vi "Set Options.vi"(8 "error in (no error)":errorcluster, 10 "UI Options":T1, 11 "FormulaG API in":refnum<class "FormulaG API.lvclass">) -> (0 "error out":errorcluster, 3 "FormulaG API out":refnum<class "FormulaG API.lvclass">)   [LabVIEW 2020, in "FormulaG.lvlib" / "FormulaG API.lvclass"]
uses:
  FormulaG API.lvclass
  FormulaG-Common/UI Options.ctl
  Command.ctl
  FormulaG API.lvclass/FormulaG API.ctl
  <vilib>/IlluminatedG/IG GodotServer/GodotLV/GodotServer/GodotServer.lvclass
  FormulaG-Common/FormulaG-Common.lvlib
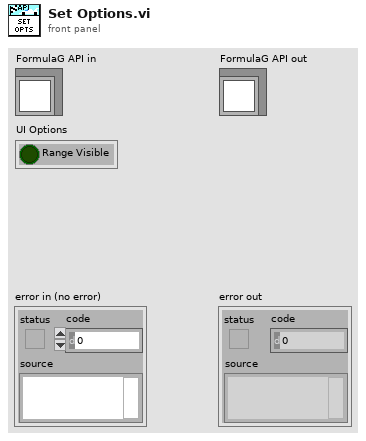
[diagram p1: front panel]
types:
  T1 = typedef "FormulaG-Common.lvlib/UI Options.ctl" = cluster{"Range Visible":bool}
  T2 = enum16{"big-endian, network order", "native, host order", "little-endian"}
  T3 = typedef "FormulaG.lvlib/FormulaG API.lvclass/Command.ctl" = enum8{"None", "Reset Car", "Request State", "Control Car", "Request Info", "Set Options", "Set Camera", "Set Pause", "Request Time"}
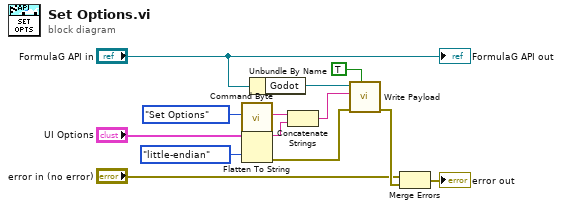
[diagram p0: block diagram]
diagram:
  n1 = call "Command Byte.vi"("Command"=Command."Set Options") -> ("Command Byte"=w12:string)  [unwired: 10 in]
  n2 = Flatten To String(anything="UI Options", byte order (0:big-endian, network order)=T2."little-endian") -> (data string=w4:string, error out=w2:errorcluster)  [unwired: 2 in, 1 out]
  n3 = Unbundle By Name("FormulaG API in") -> ("Godot"=w11:refnum<class "GodotServer.lvclass">)
  n4 = Concatenate Strings(w12, w4) -> (w10:string)
  n5 = call <vilib>:"Write Payload.vi"("Binary (F = Text)"=TRUE, "error in (no error)"=w2, "Payload"=w10, "GodotServer in"=w11) -> ("error out"=w8:errorcluster)  [unwired: 6 in, 1 out]
  n6 = Merge Errors("error in (no error)", w8) -> (→"error out":errorcluster)
  "FormulaG API out" <- "FormulaG API in"
